vi "Abort trigger.vi"(8 "error in (no error)":errorcluster, 9 "Timed out waiting on data":bool, 10 "Logging queue element in":T2 {"Ref Dwell time (us)" format="%#.6g"; "Frame Size" items=["100X100"=100, "128X128"=128, "200X200"=200, "256X256"=256, "512X512"=512, "1024x1024"=1024, "2048x2048"=2048]; "Dwell time (us)" format="%#.6g"}, 11 "Logging queue in":T1) -> (0 "error out":errorcluster, 1 "Stop the acquisition module":bool, 2 "Logging queue metadata shift out":T2 {"Ref Dwell time (us)" format="%#.6g"; "Frame Size" items=["100X100"=100, "128X128"=128, "200X200"=200, "256X256"=256, "512X512"=512, "1024x1024"=1024, "2048x2048"=2048]; "Dwell time (us)" format="%#.6g"}, 3 "Logging queue out":T1)   [LabVIEW 2020]
uses:
  Typedefs/Logging queue element.ctl
  Typedefs/Imaging Protocols enum.ctl
  Typedefs/Frame Size.ctl
  Typedefs/Acquired points count.ctl
  Typedefs/Data queue ref.ctl
  Typedefs/Read Write Enum.ctl
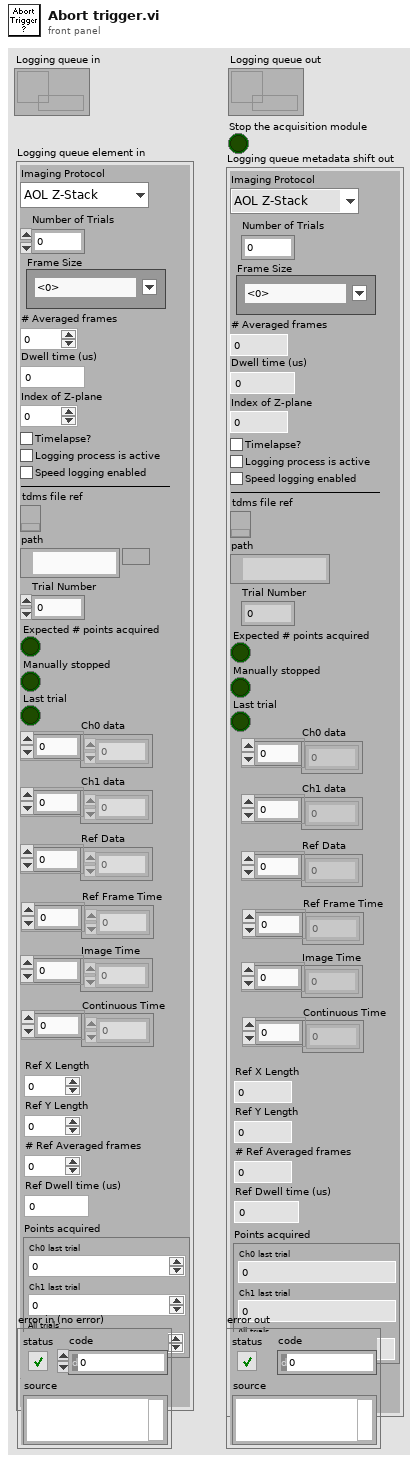
[diagram p1: front panel]
types:
  T1 = typedef "Data queue ref.ctl" = refnum<queue>
  T2 = typedef "Logging queue element.ctl" = cluster{"Imaging Protocol":T3, "Number of Trials":u16, "Frame Size":T4, "# Averaged frames":u16, "Dwell time (us)":dbl, "Index of Z-plane":i32, "Timelapse?":bool, "Logging process is active":bool, "Speed logging enabled":bool, "tdms file ref":refnum<k34>, "path":path, "Trial Number":i32, "Expected # points acquired":bool, "Manually stopped":bool, "Last trial":bool, "Ch0 data":u32[], "Ch1 data":u32[], "Ref Data":u32[], "Ref Frame Time":u64[], "Image Time":u64[], "Continuous Time":u64[], "Ref X Length":u16, "Ref Y Length":u16, "# Ref Averaged frames":u16, "Ref Dwell time (us)":dbl, "Points acquired":T5, "HW Timings File":refnum<file>}
  T3 = typedef "Imaging Protocols enum.ctl" = enum16{"AOL Z-Stack", "Motor Z Stack", "Functional Acquisition", "Single Plane Acquisition", "Volume Acquisition", "Live Imaging", "Live Plane Imaging", "Live Volume Imaging"}
  T4 = typedef "Frame Size.ctl" = u16
  T5 = typedef "Acquired points count.ctl" = cluster{"Ch0 last trial":u64, "Ch1 last trial":u64, "All trials":u64}
  T6 = typedef "Read Write Enum.ctl" = enum16{"Read", "Write"}
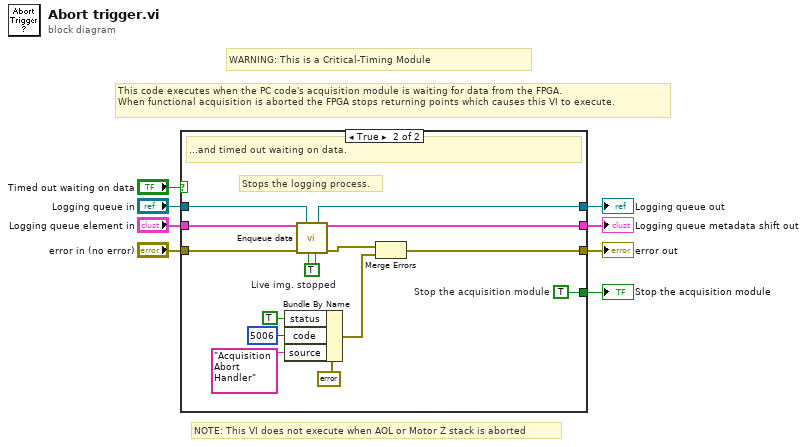
[diagram p0: block diagram]
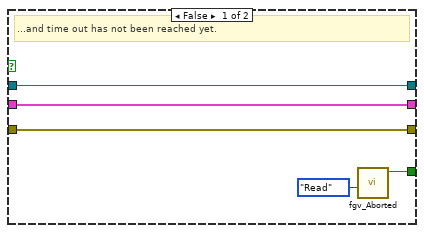
[diagram p2: hidden frame]
diagram:
  # "NOTE: This VI does not execute when AOL or Motor Z stack is aborted"
  # "WARNING: This is a Critical-Timing Module"
  # "This code executes when the PC code's acquisition module is waiting for data from the FPGA.\nWhen functional acquisition is aborted the FPGA stops returning points which causes this VI to execute."
  n1 = case shown="True" "Timed out waiting on data" {
    tunnel: [w13 w19] -> w3
    tunnel: "error in (no error)" -> [w13 w23]
    tunnel: "Logging queue in" -> [w12 w16]
    tunnel: "Logging queue element in" -> [w11 w17]
    tunnel: [w12 w15] -> w6
    tunnel: [w11 w18] -> w8
    tunnel: [w9 w14] -> w1
    frame False {
      # "...and time out has not been reached yet."
      n2 = call "fgv_Aborted.vi"("Function"=Read_Write_Enum."Read") -> ("Funct Acq Aborted?"=w9:bool)  [unwired: 9 in, 1 out]
    }
    frame True {
      w14 = TRUE  # Stop the acquisition module
      w24 = TRUE  # Live img. stopped
      # "Stops the logging process."
      # "...and timed out waiting on data."
      n3 = Bundle By Name(cluster=errorcluster {"status"=FALSE, "code"=0, "source"=""} ("error out"), "status"=TRUE, "code"=5006, "source"="Acquisition Abort Handler") -> (w21:errorcluster)
      n4 = call "Enqueue data.vi"("Logging queue metadata shift in"=w17, "Logging queue in"=w16, "Error in"=w23, "Expected # points acquired"=w24, "Manually stopped"=w24) -> ("Logging queue out"=w15:T1, "Logging queue metadata shift out"=w18:T2, "error out"=w22:errorcluster)  [unwired: 8 in]
      n5 = Merge Errors(w22, w21) -> (w19:errorcluster)
    }
  }
  "Logging queue metadata shift out" <- w8
  "Logging queue out" <- w6
  "error out" <- w3
  "Stop the acquisition module" <- w1
